vi "Execute Command.vi"(8 "error in (no error)":errorcluster, 10 "command":T1={"Command"=enum."Rx", "Parameters"={"arg1"=0, "arg2"=0}}, 11 "Dispatcher in":refnum<class "Dispatcher Thread.lvclass">) -> (0 "error out":errorcluster, 3 "Dispatcher out":refnum<class "Dispatcher Thread.lvclass">)   [LabVIEW 2017, in "DSF Core.lvlib" / "Dispatcher Thread.lvclass"]
uses:
  Dispatcher Thread.lvclass
  Interface/Dispatcher/Command Data.ctl
  Interface/Dispatcher/Command.ctl
  Interface/Dispatcher/Parameters.ctl
  Dispatcher Thread.lvclass/Dispatcher Thread.ctl
  Interface/Interface.lvclass/Interface.ctl
  Interface/Logging/Send.vi
  Interface/Logging/Send Logging Command.vi
  Interface/Send Command.vi
  Interface/Write RT FIFO.vi
  Interface/Logging/Logging Interface.lvclass
  C:/Git/DSF/Core/Classes/Interface/Interface.lvclass
  VIs/VI Name.vi
  Interface/Errors.vi
  Interface/Dispatcher/Command Timeout.vi
  Interface/Dispatcher/Dispatcher Interface.lvclass
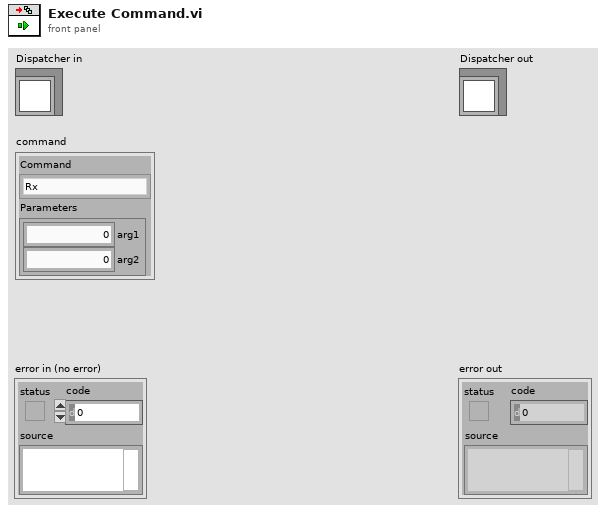
[diagram p1: front panel]
types:
  T1 = typedef "DSF Core.lvlib/Dispatcher Interface.lvclass/Command Data.ctl" = cluster{"Command":T2, "Parameters":T3}
  T2 = typedef "DSF Core.lvlib/Dispatcher Interface.lvclass/Command.ctl" = enum8{"Start", "Rx", "Tx", "Set Inline Buffer", "Shutdown"}
  T3 = typedef "DSF Core.lvlib/Dispatcher Interface.lvclass/Parameters.ctl" = cluster{"arg1":u64, "arg2":u64}
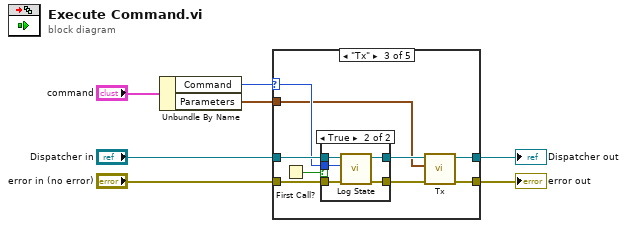
[diagram p0: block diagram]
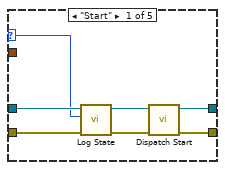
[diagram p2: hidden frame]
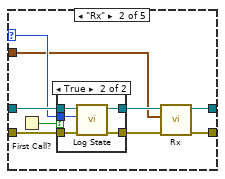
[diagram p3: hidden frame]
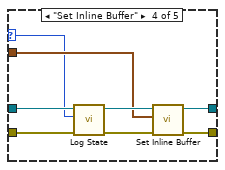
[diagram p6: hidden frame]
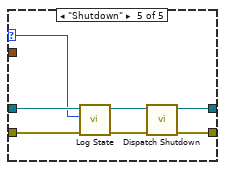
[diagram p7: hidden frame]
diagram:
  n1 = Unbundle By Name("command") -> ("Command"=w2:T2, "Parameters"=w1:T3)
  n2 = case shown="\"Tx\"" w2 {
    selector: w2 -> [w8 w16 w32 w48 w55]
    tunnel: "Dispatcher in" -> [w11 w19 w35 w52 w59]
    tunnel: [w14 w23 w39 w54 w61] -> w6
    tunnel: "error in (no error)" -> [w12 w20 w36 w51 w58]
    tunnel: [w13 w22 w38 w53 w60] -> w5
    tunnel: w1 -> [_ w15 w31 w49 _]
    frame "Start" {
      n3 = call "Log State.vi"("error in (no error)"=w12, "state"=w8, "Dispatcher in"=w11) -> ("error out"=w9:errorcluster, "Dispatcher out"=w10:refnum<class "Dispatcher Thread.lvclass">)  [unwired: 7 in]
      n4 = call "Dispatch Start.vi"("error in (no error)"=w9, "Dispatcher in"=w10) -> ("error out"=w13:errorcluster, "Dispatcher out"=w14:refnum<class "Dispatcher Thread.lvclass">)  [unwired: 8 in]
    }
    frame "Rx" {
      n5 = First Call?() -> (First Call?: T/F=w21:bool)
      n6 = case shown="True" w21 {
        tunnel: w19 -> [w25 w30]
        tunnel: w20 -> [w24 w29]
        tunnel: [w25 w28] -> w17
        tunnel: [w24 w27] -> w18
        tunnel: w16 -> [_ w26]
        frame False {
        }
        frame True {
          n7 = call "Log State.vi"("error in (no error)"=w29, "state"=w26, "Dispatcher in"=w30) -> ("error out"=w27:errorcluster, "Dispatcher out"=w28:refnum<class "Dispatcher Thread.lvclass">)  [unwired: 7 in]
        }
      }
      n8 = call "Rx.vi"("error in (no error)"=w18, "Command Parameters"=w15, "Dispatcher in"=w17) -> ("error out"=w22:errorcluster, "Dispatcher out"=w23:refnum<class "Dispatcher Thread.lvclass">)  [unwired: 7 in]
    }
    frame "Tx" {
      n9 = First Call?() -> (First Call?: T/F=w37:bool)
      n10 = case shown="True" w37 {
        tunnel: w35 -> [w41 w46]
        tunnel: w36 -> [w40 w45]
        tunnel: [w41 w44] -> w33
        tunnel: [w40 w43] -> w34
        tunnel: w32 -> [_ w42]
        frame False {
        }
        frame True {
          n11 = call "Log State.vi"("error in (no error)"=w45, "state"=w42, "Dispatcher in"=w46) -> ("error out"=w43:errorcluster, "Dispatcher out"=w44:refnum<class "Dispatcher Thread.lvclass">)  [unwired: 7 in]
        }
      }
      n12 = call "Tx.vi"("error in (no error)"=w34, "Command Parameters"=w31, "Dispatcher in"=w33) -> ("error out"=w38:errorcluster, "Dispatcher out"=w39:refnum<class "Dispatcher Thread.lvclass">)  [unwired: 7 in]
    }
    frame "Set Inline Buffer" {
      n13 = call "Log State.vi"("error in (no error)"=w51, "state"=w48, "Dispatcher in"=w52) -> ("error out"=w47:errorcluster, "Dispatcher out"=w50:refnum<class "Dispatcher Thread.lvclass">)  [unwired: 7 in]
      n14 = call "Set Inline Buffer.vi"("error in (no error)"=w47, "Command Parameters"=w49, "Dispatcher in"=w50) -> ("error out"=w53:errorcluster, "Dispatcher out"=w54:refnum<class "Dispatcher Thread.lvclass">)  [unwired: 7 in]
    }
    frame "Shutdown" {
      n15 = call "Log State.vi"("error in (no error)"=w58, "state"=w55, "Dispatcher in"=w59) -> ("error out"=w56:errorcluster, "Dispatcher out"=w57:refnum<class "Dispatcher Thread.lvclass">)  [unwired: 7 in]
      n16 = call "Dispatch Shutdown.vi"("error in (no error)"=w56, "Dispatcher in"=w57) -> ("error out"=w60:errorcluster, "Dispatcher out"=w61:refnum<class "Dispatcher Thread.lvclass">)  [unwired: 8 in]
    }
  }
  "error out" <- w5
  "Dispatcher out" <- w6
